vi "Sort.vi"(11 "strings in":T1) -> (3 "sorted strings out":T1)   [LabVIEW 2023]
uses:
  <extravilib>/ChannelInstances/Stream-str/)Channel.ctl
  <extravilib>/ChannelInstances/Stream-str/Read.vi
  <extravilib>/ChannelInstances/Stream-str/Write.vi
  <extravilib>/ChannelInstances/Stream-str/Read With Abort.vi
  <extravilib>/ChannelInstances/Stream-str/Write With Abort.vi
  <extravilib>/ChannelInstances/Stream-str/EndpointRead.vi
  <extravilib>/ChannelInstances/Stream-str/Endpoint.vi
  <extravilib>/ChannelInstances/Stream-str/)Channel.vi
  <resource>/ChannelSupport/_ChannelSupport/WaitIfNeeded.vi
  <extravilib>/ChannelInstances/Stream-str.lvlib
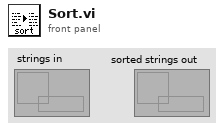
[diagram p1: front panel]
types:
  T1 = typedef "Stream-str.lvlib/)Channel.ctl" = refnum<queue>
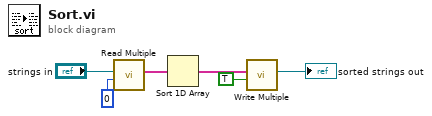
[diagram p0: block diagram]
diagram:
  n1 = call <extravilib>:"Read Multiple.vi"("number to read (-1, available)"=0, "channel"="strings in") -> ("elements"=w5:string[])  [unwired: 6 in, 3 out]
  n2 = Sort 1D Array(array=w5) -> (sorted array=w4:string[])
  n3 = call <extravilib>:"Write Multiple.vi"("last element? (F)"=TRUE ("sentinel?"), "elements"=w4) -> ("channel"=→"sorted strings out":T1)  [unwired: 6 in, 3 out]
